vi "Get FileGlobals.vi"(8 "error in (no error)":errorcluster, 11 "Session Handle in":T2) -> (0 "error out":errorcluster, 2 "FileGlobals":T1, 3 "Session Handle out":T2)   [LabVIEW 2020, in "HTS.lvlib" / "SequenceFile.lvclass"]
uses:
  SequenceFile.lvclass
  Typedefs/Session Handle.ctl
  VariableContainer/Typedefs/Session Handle.ctl
  VariableContainer/VariableContainer.lvclass
  SequenceFile.lvclass/SequenceFile.ctl
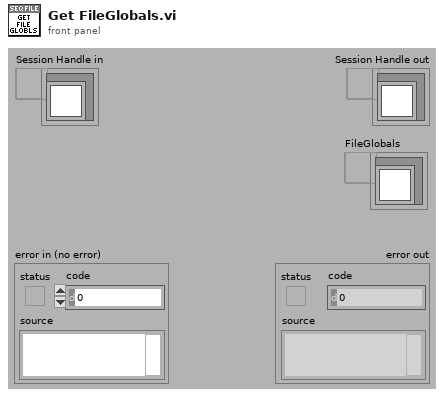
[diagram p1: front panel]
types:
  T1 = typedef "HTS.lvlib/VariableContainer.lvclass/Session Handle.ctl" = refnum<data-value>
  T2 = typedef "HTS.lvlib/SequenceFile.lvclass/Session Handle.ctl" = refnum<data-value>
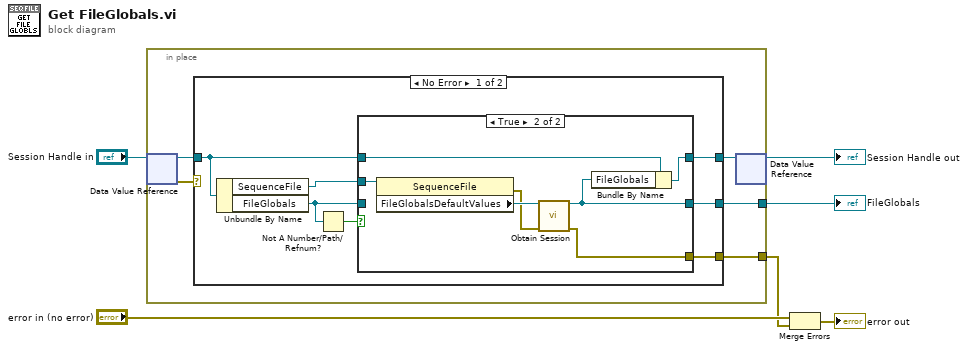
[diagram p0: block diagram]
diagram:
  n1 = in-place {
    in-place-border: [w9] -> w3
    in-place-border: [w7] -> w1
    n2 = in-place-dvr #1("Session Handle in") -> (w10:refnum<class "SequenceFile.lvclass">, w11:errorcluster)
    n3 = case shown="No Error" w11 {
      selector: w11 -> [_ w28]
      tunnel: w10 -> [w14 w29]
      tunnel: [w17 _] -> w9
      tunnel: [w13 w29] -> w8
      tunnel: [w12 w28] -> w7
      frame No Error {
        n4 = Unbundle By Name(w14) -> ("SequenceFile"=w18:refnum<k7>, "FileGlobals"=w15:T1)
        n5 = Not A Number/Path/Refnum?(number/path/refnum=w15) -> (NaN/Path/Refnum?=w16:bool)
        n6 = case shown="True" w16 {
          tunnel: w18 -> [_ w27]
          tunnel: [w19 w24] -> w17
          tunnel: w15 -> [w19 _]
          tunnel: w14 -> [w20 w25]
          tunnel: [w20 w23] -> w13
          tunnel: [_ w21] -> w12
          frame False {
            # "Already session'd - simple return"
          }
          frame True {
            n7 = property class="SequenceFile"(reference=w27) -> (error out=w22:errorcluster, "FileGlobalsDefaultValues"=w26:refnum<k7>)  [unwired: 1 in, 1 out]
            n8 = call "Obtain Session.vi"("PropertyObject"=w26, "error in (no error)"=w22) -> ("Session Handle"=w24:T1, "error out"=w21:errorcluster)  [unwired: 12 in]
            n9 = Bundle By Name(cluster=w25, "FileGlobals"=w24) -> (w23:refnum<class "SequenceFile.lvclass">)
          }
        }
      }
      frame Error {
      }
    }
    n10 = in-place-dvr #1(w8) -> (→"Session Handle out":T2)  [unwired: 1 out]
  }
  "FileGlobals" <- w3
  n11 = Merge Errors("error in (no error)", w1) -> (→"error out":errorcluster)
